vi "calcActForce.vi"() -> ()   [LabVIEW 2016]
uses:
  BendModeToForce/BendModeToForce.lvclass
panel:
  out "Transformed Mirror DOF (um)":dbl[](array[numeric])
  in  "Configuration":T1={"Config Dir"=path "/home/ttsai/Documents/stash/ts_tcs_ofc/configData", "Bending Mode Files"={"M1M3 Subsystem"={"Mirror"="M1M3", "Actuatro Force File"="M1M3_1um_156_force.txt"}, "M2 Subsystem"={"Mirror"="M2", "Actuatro Force File"="M2_1um_force.DAT"}, "Num of Bending Mode"=20}, "Rot Mirror FEA File Name"="rotMat_Bo_to_Chris_FEA_DOF.txt"}
  out "Actuator Force (N)":dbl[](array[numeric])
  in  "Mirror DOF (um)":dbl[](array[numeric])=[0.0, 0.0, 0.0, 0.0, 0.0, 0.0, 0.0, 0.0, 0.0, 0.0, 0.0, 0.0, 0.0, 0.0, 0.0, 0.0, 0.0, 0.0, 0.0, 0.0]
  in  "Mirror":enum16{"M1M3", "M2"}(ring)
  in  "BendModeToForce.lvclass":refnum<class "BendModeToForce.lvclass">
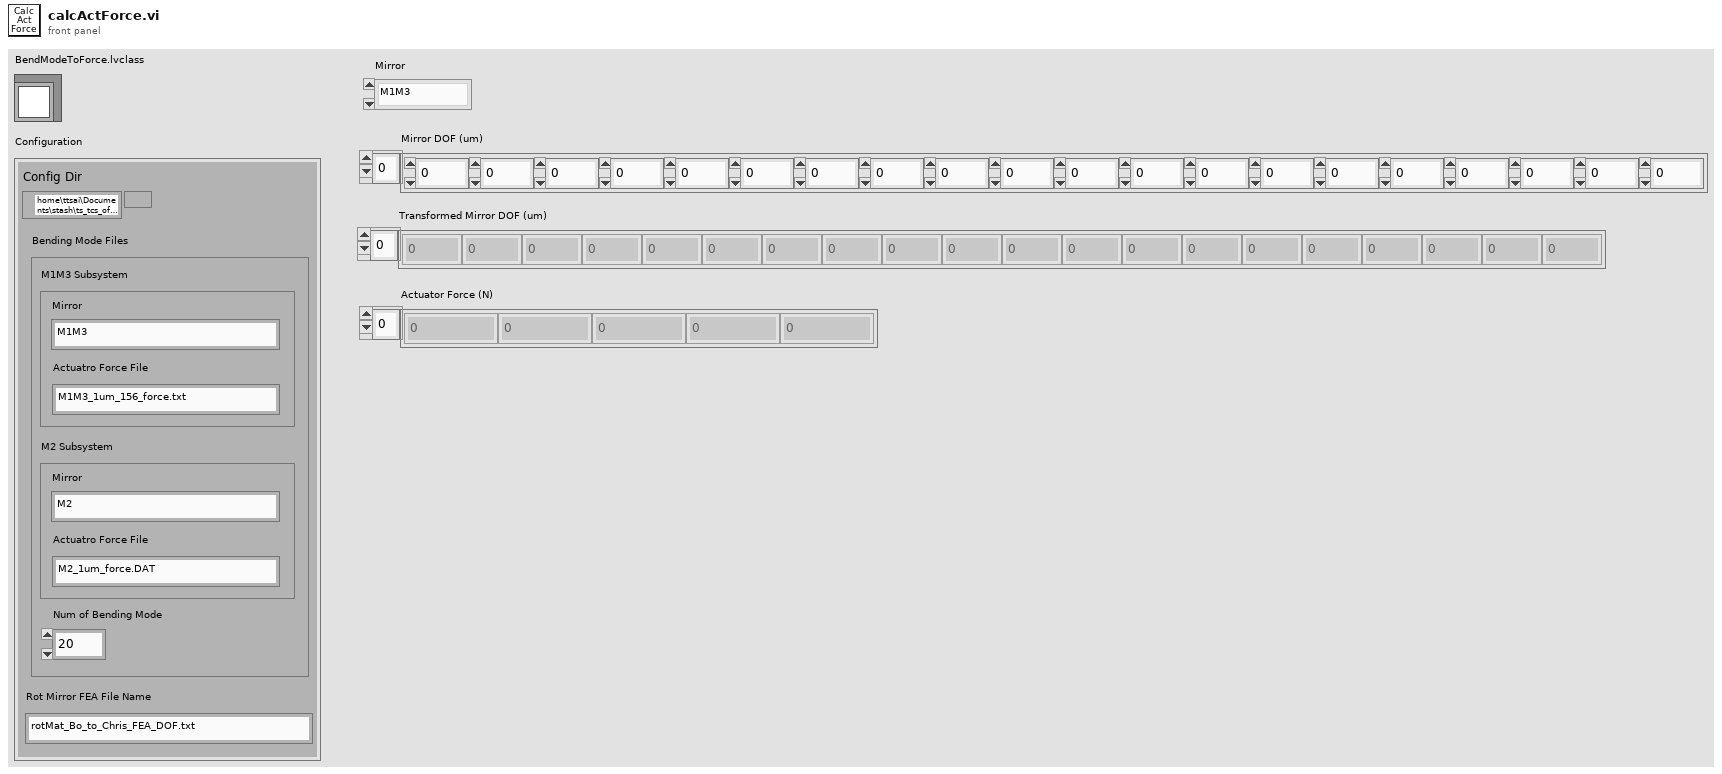
[diagram p1: front panel]
types:
  T1 = cluster{"Config Dir":path, "Bending Mode Files":cluster{"M1M3 Subsystem":cluster{"Mirror":string, "Actuatro Force File":string}, "M2 Subsystem":cluster{"Mirror":string, "Actuatro Force File":string}, "Num of Bending Mode":i32}, "Rot Mirror FEA File Name":string}
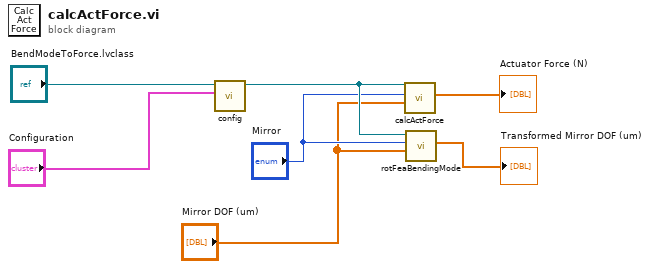
[diagram p0: block diagram]
diagram:
  n1 = call "config.vi"("Configuration"="Configuration", "BendModeToForce in"="BendModeToForce.lvclass") -> ("BendModeToForce out"=w4:refnum<class "BendModeToForce.lvclass">)  [unwired: 8 in, 1 out]
  n2 = call "calcActForce.vi"("Mirror DOF (um)"="Mirror DOF (um)", "Mirror"="Mirror", "BendModeToForce in"=w4) -> ("Actuator Force (N)"=→"Actuator Force (N)":dbl[])  [unwired: 6 in, 2 out]
  n3 = call "rotFeaBendingMode.vi"("Mirror DOF (um)"="Mirror DOF (um)", "Mirror"="Mirror", "BendModeToForce in"=w4) -> ("Transformed Mirror DOF (um)"=→"Transformed Mirror DOF (um)":dbl[])  [unwired: 6 in, 2 out]
